vi "LVClass_HasoData ctor EmptyData.vi"(0 "HasoData in":refnum<class "HasoData.lvclass">, 11 "error in (no error)":errorcluster) -> (4 "HasoData out":refnum<class "HasoData.lvclass">, 15 "error out":errorcluster)   [LabVIEW 2020, in "HasoData.lvclass"]
doc: "HasoData constructor from HasoSlopes.\n\n--------------------------------------------------------------------------------\n\n<B>HasoDataIn </B> : Constant Pointer to HasoData object.\n<B>HasoDataOut </B> : Constant Pointer to HasoData object.\n<B>HasoSlopes </B> : HasoSlopes object.\n<B>ErrorIn </B> : Error\n<B>ErrorOut </B> : Error\n\n--------------------------------------------------------------------------------"
uses:
  HasoData.lvclass
  Controls/Handle creation.ctl
  HasoData.lvclass/HasoData.ctl
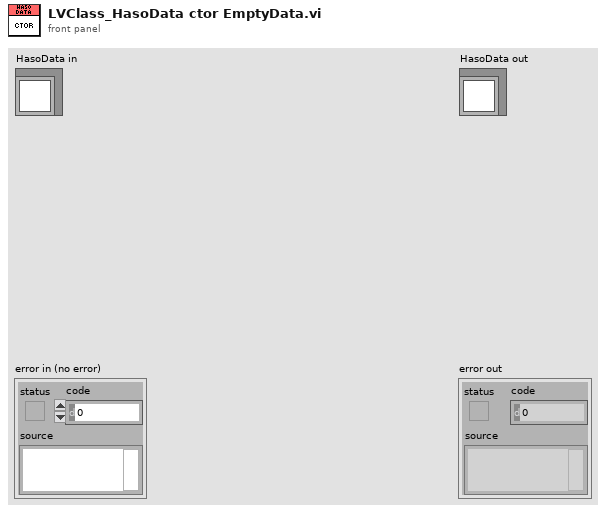
[diagram p1: front panel]
types:
  T1 = typedef "Handle creation.ctl" = enum16{"By ctor", "By write function"}
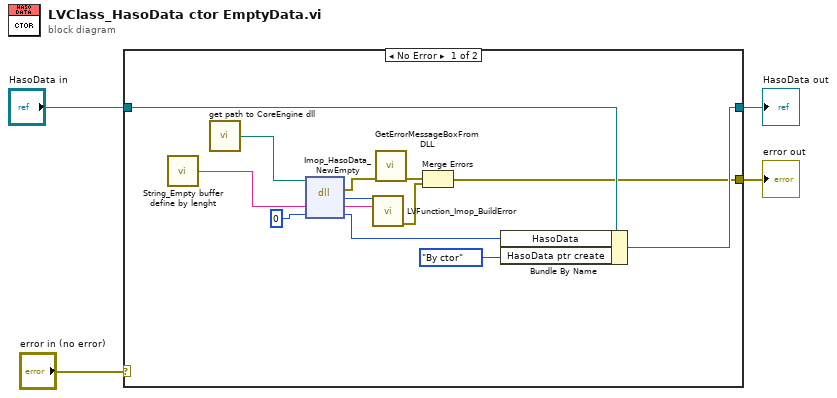
[diagram p0: block diagram]
diagram:
  n1 = case shown="No Error" "error in (no error)" {
    selector: "error in (no error)" -> [_ w19]
    tunnel: [w5 w19] -> w2
    tunnel: [w11 w18] -> w1
    tunnel: "HasoData in" -> [w12 w18]
    frame No Error {
      n2 = call "String_Empty buffer define by lenght.vi"() -> ("Empty buffer"=w13:string)  [unwired: 1 in]
      n3 = call "get path to CoreEngine dll.vi"() -> ("path to wavekit library"=w10:path)  [unwired: 14 in, 1 out]
      n4 = dll-call lib="D:/soft/HASO_v3/SVN_trunk/ImOpCoreEngine4_LV2011/DLLs/c_interface_vc100.dll" fn="Imop_HasoData_NewEmpty"(path in=w10, "message"=w13, "objet"=0) -> (error out=w9:errorcluster, "return type"=w16:i32, "message"=w15:string, "objet"=w14:i64)  [unwired: 2 in, 1 out]
      n5 = call "LVFunction_Imop_BuildError.vi"("code"=w16, "String to Prepend to source (\"\")"=w15) -> ("error out"=w6:errorcluster)  [unwired: 13 in]
      n6 = call "GetErrorMessageBoxFromDLL.vi"("error IN"=w9) -> ("error OUT"=w7:errorcluster)  [unwired: 10 in]
      n7 = Merge Errors(w7, w6) -> (w5:errorcluster)
      n8 = Bundle By Name(cluster=w12, "HasoData"=w14, "HasoData ptr create"=Handle_creation."By ctor") -> (w11:refnum<class "HasoData.lvclass">)
    }
    frame Error {
    }
  }
  "error out" <- w2
  "HasoData out" <- w1
